vi "HFRR ADV v016 new software.vi"() -> ()   [LabVIEW 2025] (continued)
                n3061 = local write "Numeric 10"(w4047) -> ()
              }
              frame #1 {
                n3062 = local read "S.NO"() -> (→"s.NO":string)
                n3063 = local read "String 29"() -> (w4051:string)
                n3064 = String To Path(string=w4051) -> (path=w4050:path)
                n3065 = Open/Create/Replace File "Open File"(file path (use dialog)=w4050) -> (refnum out=w4052:refnum<file>)  [unwired: 5 in, 2 out]
                n3066 = for {
                  N: 16 -> [_]
                  tunnel: w4052 -> [w4059]
                  i -> [w4055]
                  (unwired) TRUE ("line mode (F)")
                  n3067 = Read from Text File "Read File"(file (use dialog)=w4059) -> (text=w4053:string)  [unwired: 3 in, 3 out]
                  n3068 = Match Pattern(string=w4053, regular expression="(") -> (after substring=w4058:string)  [unwired: 1 in, 3 out]
                  n3069 = Match Pattern(string=w4058, regular expression=")") -> (before substring=w4054:string)  [unwired: 1 in, 3 out]
                  n3070 = case shown="1" w4055 {
                    tunnel: w4054 -> [w4060 w4061 _ _ w4062 w4063 w4064 w4066 w4068 w4070 w4072 w4074 w4076 w4078 _]
                    tunnel: w4053 -> [_ _ _ _ _ _ _ _ _ _ _ _ _ _ _]
                    frame 0 {
                      "TITTLE" <- w4060
                    }
                    frame 1 {
                      "Sample ID" <- w4061
                    }
                    frame 2 {
                    }
                    frame 3 {
                    }
                    frame 4 {
                      "Test Date" <- w4062
                    }
                    frame 5 {
                      "Tested by" <- w4063
                    }
                    frame 6 {
                      n3071 = Fract/Exp String To Number(string=w4064) -> (number=→"Humidity before test 2":dbl)  [unwired: 3 in, 1 out]
                    }
                    frame 7 {
                      n3072 = Fract/Exp String To Number(string=w4066) -> (number=→"Temperature before test 2":dbl)  [unwired: 3 in, 1 out]
                    }
                    frame 8 {
                      n3073 = Fract/Exp String To Number(string=w4068) -> (number=→"Humidity after test 2":dbl)  [unwired: 3 in, 1 out]
                    }
                    frame 9 {
                      n3074 = Fract/Exp String To Number(string=w4070) -> (number=→"Temperature after test 2":dbl)  [unwired: 3 in, 1 out]
                    }
                    frame 10 {
                      n3075 = Fract/Exp String To Number(string=w4072) -> (number=→"MWSD 2":dbl)  [unwired: 3 in, 1 out]
                    }
                    frame 11 {
                      n3076 = Fract/Exp String To Number(string=w4074) -> (number=→"AVP 2":dbl)  [unwired: 3 in, 1 out]
                    }
                    frame 12 {
                      n3077 = Fract/Exp String To Number(string=w4076) -> (number=→"HCF 2":dbl)  [unwired: 3 in, 1 out]
                    }
                    frame 13 {
                      n3078 = Fract/Exp String To Number(string=w4078) -> (number=→"WS1.4 2":dbl)  [unwired: 3 in, 1 out]
                    }
                    frame 14, Default {
                    }
                  }
                }
              }
              frame #2 {
              }
            }
            n3079 = local write "OK Button 16"(FALSE ("OK Button 13")) -> ()
          }
        }
        n3080 = Index Array(array=w3722, index="Select Printer 3") -> (element=w3724:string)
        "Selected Printer" <- w3724
        n3081 = case shown="True" w3719 {
          frame False {
          }
          frame True {
            n3082 = flat-sequence {
              frame #0 {
              }
              frame #1 {
                n3083 = Wait (ms)(milliseconds to wait=u32 100) -> ()  [unwired: 1 out]
              }
              frame #2 {
                n3084 = local write "OK Button 16"(FALSE ("Print 3")) -> ()
              }
            }
          }
        }
        n3085 = case shown="True" "Print" {
          tunnel: w3724 -> [_ w4016]
          frame False {
          }
          frame True {
            (unwired) i16 6 ("width (-)")
            (unwired) "TESTED BY : "
            (unwired) "TESTED DATE :"
            (unwired) "SAMPLE ID : "
            (unwired) "SAMPLE DESIGN : "
            w3974 = "\r"
            w3991 = "\r"
            # "add image"
            n3086 = local read "Sample ID"() -> (w3964:string)
            n3087 = local read "Tested by"() -> (w3967:string)
            n3088 = local read "String 34"() -> (w3954:string)
            n3089 = local read "String 45"() -> (w3934:string)
            n3090 = local read "String 35"() -> (w3949:string)
            n3091 = local read "String 37"() -> (w3947:string)
            n3092 = local read "String 32"() -> (w3969:string)
            n3093 = local read "String 36"() -> (w3944:string)
            n3094 = local read "String 31"() -> (w3968:string)
            n3095 = local read "Test Date"() -> (w3965:string)
            n3096 = local read "String 33"() -> (w3970:string)
            n3097 = local read "String 38"() -> (w3940:string)
            n3098 = local read "String 39"() -> (w3937:string)
            n3099 = local write "Print"(FALSE ("Print FF")) -> ()
            n3100 = local read "S 39"() -> (w3952:string)
            n3101 = local read "S 38"() -> (w3959:string)
            n3102 = local read "Temperature before test 2"() -> (w3990:dbl)
            n3103 = local read "Temperature after test 2"() -> (w3980:dbl)
            n3104 = local read "Humidity before test 2"() -> (w4005:dbl)
            n3105 = local read "Humidity after test 2"() -> (w3989:dbl)
            n3106 = local read "MWSD 2"() -> (w3994:dbl)
            n3107 = local read "WS1.4 2"() -> (w3972:dbl)
            n3108 = Concatenate Strings("2)" ("string"), w3954) -> (w3955:string)
            n3109 = Concatenate Strings("3)" ("string"), w3952) -> (w3953:string)
            n3110 = Concatenate Strings("1)" ("string"), w3959) -> (w3958:string)
            n3111 = Concatenate Strings("4)" ("string"), w3949) -> (w3950:string)
            n3112 = Concatenate Strings("5)" ("string"), w3947) -> (w3946:string)
            n3113 = Concatenate Strings("6)" ("string"), w3944) -> (w3943:string)
            n3114 = Concatenate Strings("7)" ("string"), w3940) -> (w3941:string)
            n3115 = Concatenate Strings("8)" ("string"), w3937) -> (w3938:string)
            n3116 = local read "HCF 2"() -> (w3976:dbl)
            n3117 = local read "AVP 2"() -> (w3993:dbl)
            n3118 = local read "s.NO"() -> (w3935:string)
            n3119 = call <vilib>:"New Report.vi"("report type"=enum16{"Standard Report", "HTML"}."Standard Report") -> ("report out"=w4014:refnum<class "NI_report.lvclass">, "error out"=w4013:errorcluster)  [unwired: 13 in]
            n3120 = local read "TITTLE"() -> (w3966:string)
            n3121 = Concatenate Strings(w3991, w3934, w3935, w3991, w3969, w3964, w3991, w3968, w3965, w3991, w3970, w3967, w3991) -> (w3984:string)
            "test by" <- w3984
            n3122 = Number To Fractional String(number=w3990, width (-)=i16 6, precision (6)=i16 2) -> (F-format string=w3979:string)  [unwired: 1 in]
            n3123 = Number To Fractional String(number=w3989, width (-)=i16 6, precision (6)=i16 2) -> (F-format string=w3992:string)  [unwired: 1 in]
            n3124 = Number To Fractional String(number=w4005, width (-)=i16 6, precision (6)=i16 2) -> (F-format string=w4010:string)  [unwired: 1 in]
            n3125 = Number To Fractional String(number=w3994, width (-)=i16 6, precision (6)=i16 2) -> (F-format string=w3996:string)  [unwired: 1 in]
            n3126 = Number To Fractional String(number=w3980, width (-)=i16 6, precision (6)=i16 2) -> (F-format string=w3981:string)  [unwired: 1 in]
            n3127 = Number To Fractional String(number=w3993, width (-)=i16 6, precision (6)=i16 2) -> (F-format string=w3995:string)  [unwired: 1 in]
            n3128 = Number To Fractional String(number=w3976, width (-)=i16 6, precision (6)=i16 2) -> (F-format string=w3975:string)  [unwired: 1 in]
            n3129 = Number To Fractional String(number=w3972, precision (6)=i16 2) -> (F-format string=w3971:string)  [unwired: 2 in]
            n3130 = call-dynamic "Set Report Header Text.vi"("report in"=w4014, "center header text"=w3966, "error in (no error)"=w4013) -> ("report out"=w3985:refnum<class "NI_report.lvclass">, "error out"=w3986:errorcluster)  [unwired: 11 in]
            n3131 = Concatenate Strings(w3974, w3958, w4010, w3974, w3955, w3979, w3974, w3953, w3992, w3974, w3950, w3981, w3974, w3946, w3996, w3974, w3943, w3995, w3974, w3941, w3975, w3974, w3938, w3971) -> (w3962:string)
            "export 2" <- w3962
            n3132 = call-poly <vilib>:"Append Report Text.vi"("report in"=w3985, "text"=w3984, "error in (no error)"=w3986) -> ("report out"=w3988:refnum<class "NI_report.lvclass">, "error out"=w3987:errorcluster)  [unwired: 9 in, 2 out]
            n3133 = local read "test by"() -> (w3961:string)
            n3134 = local read "TITTLE"() -> (w3963:string)
            n3135 = call-poly <vilib>:"Append Report Text.vi"("report in"=w3988, "error in (no error)"=w3987) -> ("report out"=w4009:refnum<class "NI_report.lvclass">, "error out"=w4007:errorcluster)  [unwired: 10 in, 2 out]
            n3136 = Concatenate Strings(w3963, w3962, w3961) -> (→"output":string)
            n3137 = call-poly <vilib>:"Append Report Text.vi"("report in"=w4009, "text"=w3962, "error in (no error)"=w4007) -> ("report out"=w4008:refnum<class "NI_report.lvclass">, "error out"=w4006:errorcluster)  [unwired: 9 in, 2 out]
            n3138 = call-dynamic "Print Report.vi"("report in"=w4008, "printer name (default)"=w4016, "error in (no error)"=w4006) -> ("report out"=w4018:refnum<class "NI_report.lvclass">, "error out"=w4019:errorcluster)  [unwired: 11 in]
            n3139 = call-dynamic "Dispose Report.vi"("report in"=w4018, "error in (no error)"=w4019) -> ()  [unwired: 13 in, 1 out]
          }
        }
        n3140 = case shown="True" "Print 2" {
          frame False {
          }
          frame True {
            n3141 = flat-sequence {
              frame #0 {
                n3142 = local read "s.NO"() -> (→"s.NO 2":string)
                n3143 = Wait (ms)(milliseconds to wait=u32 20) -> ()  [unwired: 1 out]
                n3144 = local read "Sample ID  3"() -> (→"Sample ID  6":string)
                n3145 = local read "Sample ID  4"() -> (→"Sample ID  7":string)
                n3146 = local read "Sample ID"() -> (→"Sample ID  2":string)
                n3147 = local read "Tested by"() -> (→"Tested by 2":string)
                n3148 = local read "Test Date"() -> (→"Test Date 2":string)
                n3149 = local read "Humidity after test 3"() -> (→"Humidity after test 4":dbl)
                n3150 = local read "Ref A Test Date :"() -> (→"TITTLE 4":string)
                n3151 = local read "Temperature before test 3"() -> (w3841:dbl)
                n3152 = local read "Temperature before test 3"() -> (→"Temperature after test 5":dbl)
                n3153 = local read "Temperature after test 3"() -> (→"Temperature after test 4":dbl)
                n3154 = local read "Humidity before test 3"() -> (→"Humidity before test 4":dbl)
                n3155 = local write "Temperature before test 3"(w3841) -> ()
                n3156 = local read "image data"() -> (w3832:T16)
                n3157 = String To Path(string="C:\\LAB-IQ\\im\\Temp_resized.jpg") -> (path=w3833:path)
                "path 2" <- w3833
                n3158 = call <vilib>:"Write JPEG File.vi"("image data"=w3832, "path to JPEG file"=w3833) -> ()  [unwired: 8 in, 2 out]
                "Ref A Test Date :" <- "Ref A Test Date :"
                "Ref B Test Date :" <- "Ref B Test Date :"
                "Ref B Scar Value :" <- "Ref B Scar Value :"
                "Ref A Scar Value :" <- "Ref A Scar Value :"
              }
              frame #1 {
                (unwired) HTML_Report_Image_Alignment."MIDDLE" ("alignment (default)")
                w3869 = u16 0 items=["portrait", "landscape"] ("orientation (portrait)")
                (unwired) HTML_Report_Image_Alignment."ABSMIDDLE" ("alignment (default)")
                (unwired) "TESTED BY : "
                (unwired) "TESTED DATE :"
                (unwired) "SAMPLE ID : "
                (unwired) "SAMPLE DESIGN : "
                w3902 = "\r"
                # "add image"
                n3159 = Wait (ms)(milliseconds to wait=u32 20) -> ()  [unwired: 1 out]
                n3160 = local read "Sample ID  2"() -> (w3895:string)
                n3161 = local read "Wear Scar X"() -> (w3867:dbl)
                "Length ( microns ) 2" <- w3867
                n3162 = local read "Wear Scar Y"() -> (w3866:dbl)
                "Wear Scar Y ( microns ) :" <- w3866
                n3163 = local read "Test Date 2"() -> (w3896:string)
                n3164 = local read "Tested by 2"() -> (w3897:string)
                n3165 = local read "String 46"() -> (w3893:string)
                n3166 = local read "String 48"() -> (w3899:string)
                n3167 = local read "String 47"() -> (w3898:string)
                n3168 = local read "String 49"() -> (w3900:string)
                n3169 = local read "String 10"() -> (w3853:string)
                n3170 = local read "s.NO 2"() -> (w3894:string)
                n3171 = Add(x=w3867, y=w3866) -> (x+y=w3865:dbl)
                n3172 = call <vilib>:"New Report.vi"("report type"=enum16{"Standard Report", "HTML"}."HTML") -> ("report out"=w3873:refnum<class "NI_report.lvclass">, "error out"=w3871:errorcluster)  [unwired: 13 in]
                n3173 = Concatenate Strings(w3902, w3893, w3894, w3902, w3899, w3895, w3902, w3898, w3896, w3902, w3900, w3897, w3902) -> (→"test by 2":string)
                n3174 = Concatenate Strings("C:\\LAB-IQ\\Data\\" ("string"), w3853, ".jpg" ("string")) -> ()  [unwired: 1 out]
                n3175 = Divide(x=w3865, y=2.0) -> (x/y=→"Mean Wear ( microns) :":dbl)
                n3176 = call-dynamic "Set Report Orientation.vi"("report in"=w3873, "orientation (portrait)"=w3869, "error in (no error)"=w3871) -> ("report out"=w3872:refnum<class "NI_report.lvclass">, "error out"=w3870:errorcluster)  [unwired: 11 in]
                n3177 = for {
                  N: 5 -> [_]
                  tunnel: w3872 -> [w3923]
                  tunnel: [w3922] -> w3851
                  tunnel: w3870 -> [w3921]
                  tunnel: [w3920] -> w3850
                  n3178 = call-dynamic "Set Report Tab Width.vi"("report in"=w3923, "error in (no error)"=w3921) -> ("report out"=w3922:refnum<class "NI_report.lvclass">, "error out"=w3920:errorcluster)  [unwired: 12 in]
                }
                n3179 = local read "TITTLE"() -> (w3868:string)
                n3180 = call-dynamic "Set Report Header Text.vi"("report in"=w3851, "center header text"=w3868, "error in (no error)"=w3850) -> ("report out"=w3889:refnum<class "NI_report.lvclass">, "error out"=w3888:errorcluster)  [unwired: 11 in]
                n3181 = for {
                  N: 1 -> [_]
                  tunnel: [w3927] -> w3875
                  tunnel: [w3926] -> w3874
                  tunnel: w3889 -> [w3925]
                  tunnel: w3888 -> [w3924]
                  n3182 = call-dynamic "New Report Line.vi"("report in"=w3925, "error in (no error)"=w3924) -> ("report out"=w3927:refnum<class "NI_report.lvclass">, "error out"=w3926:errorcluster)  [unwired: 12 in]
                }
                n3183 = for {
                  N: 2 -> [_]
                  tunnel: [w3919] -> w3881
                  tunnel: [w3918] -> w3880
                  tunnel: w3875 -> [w3917]
                  tunnel: w3874 -> [w3916]
                  n3184 = call-dynamic "New Report Line.vi"("report in"=w3917, "error in (no error)"=w3916) -> ("report out"=w3919:refnum<class "NI_report.lvclass">, "error out"=w3918:errorcluster)  [unwired: 12 in]
                }
                n3185 = for {
                  N: 25 -> [_]
                  tunnel: w3881 -> [w3915]
                  tunnel: w3880 -> [w3913]
                  tunnel: [w3914] -> w3884
                  tunnel: [w3912] -> w3883
                  n3186 = call-dynamic "Set Report Tab Width.vi"("report in"=w3915, "error in (no error)"=w3913) -> ("report out"=w3914:refnum<class "NI_report.lvclass">, "error out"=w3912:errorcluster)  [unwired: 12 in]
                }
                n3187 = control-ref of="Tab Control 9"() -> (w3879:refnum<vi>)
                n3188 = call-dynamic "Append Control Image to Report.vi"("report in"=w3884, "alignment (default)"=HTML_Report_Image_Alignment."ABSMIDDLE", "ctrl reference"=w3879, "error in (no error)"=w3883) -> ("report out"=w3878:refnum<class "NI_report.lvclass">, "error out"=w3877:errorcluster)  [unwired: 8 in, 2 out]
                n3189 = for {
                  N: 3 -> [_]
                  tunnel: [w3911] -> w3862
                  tunnel: [w3910] -> w3861
                  tunnel: w3878 -> [w3909]
                  tunnel: w3877 -> [w3908]
                  n3190 = call-dynamic "New Report Line.vi"("report in"=w3909, "error in (no error)"=w3908) -> ("report out"=w3911:refnum<class "NI_report.lvclass">, "error out"=w3910:errorcluster)  [unwired: 12 in]
                }
                n3191 = for {
                  N: 100 -> [_]
                  tunnel: w3862 -> [w3907]
                  tunnel: w3861 -> [w3905]
                  tunnel: [w3906] -> w3858
                  tunnel: [w3904] -> w3856
                  n3192 = call-dynamic "Set Report Tab Width.vi"("report in"=w3907, "error in (no error)"=w3905) -> ("report out"=w3906:refnum<class "NI_report.lvclass">, "error out"=w3904:errorcluster)  [unwired: 12 in]
                }
                n3193 = String To Path(string="C:\\LAB-IQ\\im\\Temp_resized.jpg") -> (path=w3848:path)
                n3194 = call-poly <vilib>:"Append Image to Report.vi"("report in"=w3858, "path or URL of image"=w3848, "error in (no error)"=w3856) -> ("report out"=w3857:refnum<class "NI_report.lvclass">, "error out"=w3855:errorcluster)  [unwired: 9 in, 2 out]
                n3195 = call-poly <vilib>:"Open HTML Report in Browser.vi"("report in"=w3857, "error in (no error)"=w3855) -> ("report out"=w3892:refnum<class "NI_report.lvclass">, "error out"=w3891:errorcluster)  [unwired: 11 in, 1 out]
                n3196 = call-dynamic "Dispose Report.vi"("report in"=w3892, "error in (no error)"=w3891) -> ()  [unwired: 13 in, 1 out]
              }
              frame #2 {
              }
              frame #3 {
                n3197 = disable-structure shown="Disabled" {
                  frame Disabled {
                    n3198 = local read "String 10"() -> (w3932:string)
                    n3199 = Concatenate Strings("C:\\LAB-IQ-NXT\\Data\\" ("string"), w3932, ".jpg" ("string")) -> (w3930:string)
                    n3200 = String To Path(string=w3930) -> (path=w3929:path)
                    n3201 = Delete(path (use dialog)=w3929) -> ()  [unwired: 4 in, 3 out]
                  }
                  frame Enabled {
                  }
                }
                n3202 = local write "Print 2"(FALSE ("Print")) -> ()
              }
            }
          }
        }
      }
    }
    n3203 = property on="SetTemp" class="DigNum (strict)"("Disabled"=w1868) -> ()  [unwired: 2 in, 2 out]
    n3204 = Multiply(x=w1858, y=w1860) -> (x*y=w1859:dbl)
    n3205 = local read "MWSD"() -> (w1857:dbl)
    n3206 = Add(x=w1859, y=w1857) -> (x+y=→"WS1.4":dbl)
    n3207 = Wait (ms)(milliseconds to wait=u32 50) -> ()  [unwired: 1 out]
    n3208 = Wait (ms)(milliseconds to wait=u32 50) -> ()  [unwired: 1 out]
    n3209 = local read "Quit"() -> (w1856:bool)
  }
  n3210 = VISA Close(VISA resource name=w52, error in (no error)=w51) -> (error out=w49:errorcluster)
  n3211 = call <vilib>:"Clear Errors.vi"("error in (no error)"=w49) -> ()  [unwired: 5 in, 2 out]
  n3212 = VISA Close(VISA resource name=w37, error in (no error)=w36) -> ()  [unwired: 1 out]
  n3213 = while {
    tunnel: [w4093] -> w46
    shift-right: [w4086] -> _
    shift-left: 0.0 -> [w4089]
    shift-right: [w4085] -> _
    shift-left: 0.0 -> [w4088]
    shift-right: [w4084] -> _
    shift-left: 400.0 ("vc_cmd") -> [w4087]
    stop <- w4093 stop-if-true
    # "PID LOGIC"
    n3214 = local read "RUN"() -> (w4091:bool)
    n3215 = local read "Auto Start Temp"() -> (w4080:bool)
    n3216 = local read "Auto Start Test"() -> (w4090:bool)
    n3217 = local read "START TEMP"() -> (w4082:bool)
    n3218 = And(x=w4080, y=w4090) -> (x .and. y?=w4081:bool)
    n3219 = Or(x=w4091, y=w4081) -> (x .or. y?=w4092:bool)
    n3220 = And(x=w4092, y=w4082) -> (x .and. y?=w4083:bool)
    n3221 = Wait (ms)(milliseconds to wait=u32 20) -> ()  [unwired: 1 out]
    n3222 = case shown="True" w4083 {
      tunnel: [400.0 ("out_vc_cmd") w4113] -> w4084
      tunnel: [w4096 w4115] -> w4085
      tunnel: [w4096 w4114] -> w4086
      tunnel: w4089 -> [_ w4104]
      tunnel: w4088 -> [_ w4103]
      tunnel: w4087 -> [_ w4102]
      frame False {
        w4096 = 0.0 ("error_out")
      }
      frame True {
        n3223 = local read "Set Strk"() -> (w4099:dbl)
        n3224 = local read "LVDT STROKE"() -> (w4097:dbl)
        n3225 = Add(x=w4099, y="Add up Stroke") -> (x+y=w4100:dbl)
        n3226 = formula code="// Zero-Hardcode Explicit Positional-Form PID Engine\n// Inputs: target_stroke, measured_stroke, dt, prev_error, integral_accumulator_in, prev_vc_cmd\n//         kp, ki, kd, max_step_change, max_amplitude, min_amplitude, startup_cmd\n// Outputs: vc_cmd, error_out, out_error, integral_accumulator_out, out_vc_cmd\n\n// 1. Calculate Tracking Error\nfloat current_error = target_stroke - measured_stroke;\nerror_out = current_error;\n\n// 2. Compute Proportional Term\nfloat p_term = kp * current_error;\n\n// 3. Compute Derivative Term\nfloat d_term = 0.0;\nif (dt > 0.0) {\n    d_term = kd * ((current_error - prev_error) / dt);\n}\n\n// 4. Update and Accumulate Integral Term\nfloat current_integral = integral_accumulator_in + (current_error * dt);\nfloat i_term = ki * current_integral;\n\n// 5. Calculate Ideal Target Command\nfloat ideal_command = startup_cmd + p_term + i_term + d_term;\n\n// 6. Anti-Windup Protection (Back-calculation method)\nif (ideal_command > max_amplitude) {\n    float excess = ideal_command - max_amplitude;\n    if (ki > 0.0) {\n        current_integral -= excess / ki;\n    }\n    ideal_command = max_amplitude;\n} else if (ideal_command < min_amplitude) {\n    float excess = ideal_command - min_amplitude;\n    if (ki > 0.0) {\n        current_integral -= excess / ki;\n    }\n    ideal_command = min_amplitude;\n}\n\n// 7. Apply Loop Rate Limiting (Protects voice coil from large voltage steps)\nfloat raw_adjustment = ideal_command - prev_vc_cmd;\n\nif (raw_adjustment > max_step_change) {\n    raw_adjustment = max_step_change;\n} else if (raw_adjustment < -max_step_change) {\n    raw_adjustment = -max_step_change;\n}\n\nfloat next_vc_cmd = prev_vc_cmd + raw_adjustment;\n\n// Final Output Safety Safeguard Clamping\nif (next_vc_cmd > max_amplitude) {\n    next_vc_cmd = max_amplitude;\n} else if (next_vc_cmd < min_amplitude) {\n    next_vc_cmd = min_amplitude;\n}\n\n// 8. Map to Shift Registers for memory persistence\nvc_cmd = next_vc_cmd;\nout_error = current_error;                     \nintegral_accumulator_out = current_integral;  \nout_vc_cmd = next_vc_cmd;"("target_stroke"=w4100, "measured_stroke"=w4097, "dt"="dt", "integral_accumulator_in"=w4103, "prev_error"=w4104, "prev_vc_cmd"=w4102, "kp"="kp", "ki"="ki", "kd"="kd", "max_step_change"="max_step_change", "max_amplitude"="max_amplitude", "min_amplitude"="min_amplitude", "startup_cmd"="startup_cmd") -> ("vc_cmd"=w4119:dbl, "out_error"=w4114:dbl, "integral_accumulator_out"=w4115:dbl, "out_vc_cmd"=w4113:dbl)  [unwired: 1 out]
        "output Vpp" <- w4119
        n3227 = Number To Fractional String(number=w4119, precision (6)=i16 1) -> (F-format string=w4117:string)  [unwired: 2 in]
        n3228 = Concatenate Strings("DAC;" ("string"), w4117) -> (w4101:string)
        n3229 = local write "Command"(w4101) -> ()
        "prev_error" <- w4104
        "integral_accumulator_in" <- w4103
        "prev_vc_cmd" <- w4102
      }
    }
    n3230 = local read "Quit"() -> (w4093:bool)
  }
  n3231 = Or(x=w42, y=w41) -> (x .or. y?=w43:bool)
  n3232 = Or(x=w39, y=w43) -> (x .or. y?=w48:bool)
  n3233 = control-ref of="new picture"() -> ()  [unwired: 1 out]
  n3234 = Or(x=w54, y=w48) -> (x .or. y?=w45:bool)
  n3235 = Or(x=w45, y=w46) -> (x .or. y?=w40:bool)
  n3236 = while {
    tunnel: [w4120] -> w53
    i -> [w4127]
    stop <- w4120 stop-if-true
    n3237 = local read "Quit"() -> (w4120:bool)
    n3238 = Equal To 0?(x=w4127) -> (x = 0?=w4125:bool)
    n3239 = call "Elapsed Time3"("Time Target (s)"=45.0, "Auto Reset"=TRUE) -> ("Time has Elapsed"=w4124:bool)  [unwired: 10 in, 7 out]
    n3240 = Wait (ms)(milliseconds to wait=u32 50) -> ()  [unwired: 1 out]
    n3241 = Or(x=w4124, y=w4125) -> (x .or. y?=w4126:bool)
    n3242 = case shown="True" w4126 {
      frame False {
      }
      frame True {
        n3243 = call <vilib>:"System Exec.vi"("run minimized? (F)"=TRUE, "error in (no error)"="error in (no error)", "command line"="powercfg.exe -change -monitor-timeout-ac 0") -> ("error out"=w4138:errorcluster)  [unwired: 5 in, 3 out]
        n3244 = call <vilib>:"System Exec.vi"("run minimized? (F)"=TRUE, "error in (no error)"=w4138, "command line"="powercfg.exe -change -disk-timeout-ac 0") -> ("error out"=w4137:errorcluster)  [unwired: 5 in, 3 out]
        n3245 = call <vilib>:"System Exec.vi"("run minimized? (F)"=TRUE, "error in (no error)"=w4137, "command line"="powercfg.exe -change -standby-timeout-ac 0") -> ("error out"=w4136:errorcluster)  [unwired: 5 in, 3 out]
        n3246 = call <vilib>:"System Exec.vi"("run minimized? (F)"=TRUE, "error in (no error)"=w4136, "command line"="powercfg.exe -change -hibernate-timeout-ac 0") -> ("error out"=w4135:errorcluster)  [unwired: 5 in, 3 out]
        n3247 = call <vilib>:"Simple Error Handler.vi"("error in (no error)"=w4135) -> ("error out"=w4141:errorcluster)  [unwired: 4 in, 4 out]
        n3248 = call <vilib>:"Clear Errors.vi"("error in (no error)"=w4141) -> ("error out"=→"error out":errorcluster)  [unwired: 5 in, 1 out]
      }
    }
  }
  n3249 = Compound Arithmetic op=OR(w56, w40, w53) -> (w55:bool)
  n3250 = flat-sequence {
    tunnel: w55 -> [_]
    tunnel: [w4143] -> w18
    tunnel: w18 -> [_]
    frame #0 {
      n3251 = call "CLOSE CONNECTION.vi"() -> ("error out"=w4143:errorcluster)  [unwired: 11 in]
    }
    frame #1 {
      n3252 = Quit LabVIEW(quit? (T)=TRUE) -> ()
      n3253 = local write "Quit"(FALSE ("EXIT")) -> ()
    }
  }
  n3254 = property on="Heater Button" class="Bool (strict)"("Visible"=TRUE) -> ()  [unwired: 2 in, 2 out]
  n3255 = disable-structure shown="Disabled" {
    disable-tunnel: _ -> [w4149 _]
    disable-tunnel: _ -> [w4146 _]
    disable-tunnel: _ -> [w4147 _]
    frame Disabled {
      n3256 = disable-structure shown="Disabled" {
        disable-tunnel: [w4156 _] -> w4148
        frame Disabled {
          n3257 = while {
            shift-right: [w4198] -> w4154
            shift-left: errorcluster {"status"=TRUE, "code"=0, "source"="Init"} ("error out") -> [w4163]
            shift-right: [w4197] -> w4153
            shift-left: _ -> [w4164]
            shift-right: [w4196] -> _
            shift-left: "" -> [w4195]
            tunnel: [w4157] -> w4156
            shift-right: ["Set Rh"] -> _
            shift-left: 0.0 ("Set Rh") -> [w4189]
            tunnel: [w4166] -> _
            i -> [w4166]
            stop <- w4157 stop-if-true
            n3258 = flat-sequence {
              tunnel: w4163 -> [w4201]
              tunnel: [w4201] -> w4162
              frame #0 {
                n3259 = Wait (ms)(milliseconds to wait=u32 200) -> ()  [unwired: 1 out]
              }
            }
            n3260 = local read "Com Port 3"() -> (w4165:refnum<visa-resource-name>)
            n3261 = local read "Humidity Str Rec"() -> (w4167:string)
            n3262 = Not Equal?(x="Set Rh", y=w4189) -> (x != y?=w4194:bool)
            n3263 = Number To Decimal String(number="Set Rh") -> (decimal integer string=w4192:string)  [unwired: 1 in]
            n3264 = Not Equal?(x=w4165, y=w4164) -> (x != y?=w4160:bool)
            n3265 = Concatenate Strings("#setPoint00" ("string"), w4192) -> (w4193:string)
            n3266 = case shown="False" w4194 {
              tunnel: w4193 -> [_ w4213]
              frame False {
                n3267 = local read "Humidity"() -> (w4210:bool)
                n3268 = case shown="True" w4210 {
                  frame False {
                    n3269 = local write "Humidity Str Send"("stop" ("Humidity Str Send")) -> ()
                  }
                  frame True {
                    n3270 = local write "Humidity Str Send"("start" ("Humidity Str Send")) -> ()
                  }
                }
              }
              frame True {
                n3271 = local write "Humidity Str Send"(w4213) -> ()
              }
            }
            n3272 = Or(x=w4160) -> (y=w4158:bool, x .or. y?=w4159:bool)
            n3273 = String Subset(string=w4167, offset (0)=7) -> (substring=w4182:string)  [unwired: 1 in]
            n3274 = Match Pattern(string=w4167, regular expression="?") -> (offset past match=w4185:i32)  [unwired: 1 in, 3 out]
            n3275 = Match Pattern(string=w4167, regular expression="v") -> (offset past match=w4188:i32)  [unwired: 1 in, 3 out]
            n3276 = case shown="True" w4159 {
              tunnel: w4162 -> [w4199 _]
              tunnel: [w4199 errorcluster {"status"=TRUE, "code"=0, "source"="Init"} ("error out")] -> w4161
              frame False {
              }
              frame True {
              }
            }
            n3277 = Equal?(x=w4185, y=-1) -> (x = y?=w4169:bool)
            n3278 = Match Pattern(string=w4182, regular expression="g") -> (after substring=w4183:string, offset past match=w4174:i32)  [unwired: 1 in, 2 out]
            n3279 = Match Pattern(string=w4182, regular expression="y") -> (after substring=w4181:string, offset past match=w4175:i32)  [unwired: 1 in, 2 out]
            n3280 = Greater?(x=w4175, y=w4174) -> (0:w4180:bool)
            n3281 = Greater Or Equal To 0?(x=w4175) -> (x >= 0?=w4172:bool)
            n3282 = Greater Or Equal To 0?(x=w4174) -> (x >= 0?=w4173:bool)
            n3283 = Or(x=w4172, y=w4173) -> (x .or. y?=w4171:bool)
            n3284 = Greater Or Equal To 0?(x=w4188) -> (x >= 0?=w4170:bool)
            n3285 = Select(t=w4181, s=w4180, f=w4183) -> (s? t:f=w4176:string)
            n3286 = case shown="Error" w4161 {
              selector: w4161 -> [w4226 w4272]
              tunnel: [w4224 w4265] -> w4198
              tunnel: w4164 -> [w4227 w4271]
              tunnel: [w4225 w4274] -> w4197
              tunnel: w4195 -> [w4214 w4273]
              tunnel: [w4221 w4273] -> w4196
              frame No Error {
                n3287 = call "Elapsed Time7"() -> ("Time has Elapsed"=w4220:bool)  [unwired: 12 in, 7 out]
                n3288 = Not Equal?(x="Humidity Str Send", y=w4214) -> (x != y?=w4216:bool)
                n3289 = Or(x=w4216, y=w4220) -> (x .or. y?=w4219:bool)
                n3290 = Select(t="Humidity Str Send", s=w4216, f="vals" ("regular expression")) -> (s? t:f=w4215:string)
                n3291 = Or(x=w4219, y="Send") -> (x .or. y?=w4223:bool)
                n3292 = case shown="True" w4223 {
                  tunnel: [w4230 w4235] -> w4224
                  tunnel: w4227 -> [w4229 w4243]
                  tunnel: w4226 -> [w4230 w4242]
                  tunnel: [w4229 w4236] -> w4225
                  tunnel: w4215 -> [_ w4241]
                  tunnel: [w4228 w4232] -> w4221
                  tunnel: "Humidity Str Send" -> [_ w4233]
                  tunnel: w4216 -> [_ w4234]
                  tunnel: w4214 -> [w4228 w4231]
                  frame False {
                  }
                  frame True {
                    n3293 = flat-sequence {
                      tunnel: w4243 -> [w4251]
                      tunnel: w4242 -> [w4250]
                      tunnel: w4241 -> [w4247]
                      tunnel: [w4249] -> w4240
                      tunnel: [w4248] -> w4239
                      tunnel: w4240 -> [w4254]
                      tunnel: w4239 -> [w4253]
                      tunnel: [w4254] -> w4238
                      tunnel: [w4253] -> w4237
                      tunnel: w4238 -> [w4261]
                      tunnel: w4237 -> [w4260]
                      tunnel: [w4259] -> w4236
                      tunnel: [w4258] -> w4235
                      frame #0 {
                        n3294 = local write "Ser Led"(TRUE ("Boolean 4")) -> ()
                        n3295 = Concatenate Strings(w4247, "\r") -> (w4246:string)
                        n3296 = VISA Write(VISA resource name=w4251, write buffer=w4246, error in (no error)=w4250) -> (VISA resource name out=w4249:refnum<visa-resource-name>, error out=w4248:errorcluster)  [unwired: 1 out]
                      }
                      frame #1 {
                        n3297 = Wait (ms)(milliseconds to wait="wait") -> ()  [unwired: 1 out]
                      }
                      frame #2 {
                        w4256 = FALSE ("Send")
                        n3298 = property class="Instr"(reference=w4261, error in=w4260) -> (reference out=w4262:refnum<visa-resource-name>, error out=w4263:errorcluster, "Serial Settings:Number of Bytes at Serial Port"=w4255:u32)
                        n3299 = local write "Send"(w4256) -> ()
                        n3300 = local write "Ser Led"(w4256) -> ()
                        n3301 = VISA Read(VISA resource name=w4262, byte count=w4255, error in (no error)=w4263) -> (VISA resource name out=w4259:refnum<visa-resource-name>, read buffer=→"Humidity Str Rec":string, error out=w4258:errorcluster)  [unwired: 1 out]
                      }
                    }
                    n3302 = Select(t=w4233, s=w4234, f=w4231) -> (s? t:f=w4232:string)
                  }
                }
              }
              frame Error {
                w4279 = u16 0 items=["None"=0, "XON/XOFF"=1, "RTS/CTS"=2, "DTR/DSR"=4] ("flow control")
                w4275 = u16 0 items=["None", "Odd", "Even", "Mark", "Space"] ("parity")
                w4278 = u16 10 items=["1.0"=10, "1.5"=15, "2.0"=20] ("stop bits")
                n3303 = VISA Close(VISA resource name=w4271, error in (no error)=w4272) -> (error out=w4270:errorcluster)
                n3304 = local write "humid"("" ("humid")) -> ()
                n3305 = local write "Humidity Str Rec"("" ("Humidity Str Rec")) -> ()
                n3306 = call <vilib>:"Clear Errors.vi"("error in (no error)"=w4270) -> ("error out"=w4269:errorcluster)  [unwired: 5 in, 1 out]
                n3307 = local read "Com Port 3"() -> (w4268:refnum<visa-resource-name>)
                n3308 = call-poly "VISA Configure Serial Port"("VISA resource name"=w4268, "timeout (10sec)"=u32 1000, "termination char\n(0xA = '\\n' = LF)"=u8 10 ("termination char\n(0xA = '\\n' = LF)"), "Enable Termination\nChar (T)"=FALSE ("Enable Termination Char (T)"), "data bits (8)"=u16 8 ("data bits"), "parity (0:none)"=w4275, "error in (no error)"=w4269, "stop bits (10: 1 bit)"=w4278, "flow control (0:none)"=w4279) -> ("VISA resource name out"=w4274:refnum<visa-resource-name>, "baud rate (9600)"=w4266:u32, "error out"=w4265:errorcluster)  [unwired: 4 in]
              }
            }
            n3309 = Compound Arithmetic op=AND(w4170, w4169, w4171) -> (w4168:bool)
            n3310 = case shown="True" w4168 {
              tunnel: w4167 -> [_ _]
              tunnel: w4176 -> [_ w4206]
              frame False {
              }
              frame True {
                w4204 = " " ("regular expression")
                n3311 = Match Pattern(string=w4206, regular expression=" ") -> (after substring=w4208:string)  [unwired: 1 in, 3 out]
                n3312 = Match Pattern(string=w4208, regular expression=w4204) -> (before substring=→"humid":string, after substring=w4205:string)  [unwired: 1 in, 2 out]
                n3313 = Match Pattern(string=w4205, regular expression=w4204) -> (before substring=→"temp_@Rh sensor":string)  [unwired: 1 in, 3 out]
              }
            }
            n3314 = local read "Quit"() -> (w4157:bool)
          }
          n3315 = VISA Close(VISA resource name=w4153, error in (no error)=w4154) -> (error out=w4150:errorcluster)
          n3316 = call <vilib>:"Clear Errors.vi"("error in (no error)"=w4150) -> ()  [unwired: 5 in, 2 out]
        }
        frame Enabled {
        }
      }
    }
    frame Enabled {
    }
  }
  n3317 = while {
    tunnel: [w4286] -> _
    i -> [w4286]
    stop <- w4282 stop-if-true
    # "Langauage selection"
    n3318 = Equal?(x="Lan flag", y=22.0) -> ()  [unwired: 1 out]
    n3319 = disable-structure shown="Disabled" {
      frame Disabled {
        n3320 = stacked-sequence {
          frame #0 {
            n3321 = case shown="\"Russian\"" "Language Selection" {
              tunnel: [0 1] -> w4288
              frame "English", Default {
              }
              frame "Russian" {
              }
            }
            n3322 = for {
              N: 130 -> [_]
              tunnel: "Table" -> [w4297]
              tunnel: w4288 -> [w4296]
              i -> [w4295]
              n3323 = Index Array(array=w4297, index (row)=w4295, index (col)=w4296) -> (element=w4294:string)
              n3324 = case shown="123" w4295 {
                tunnel: w4294 -> [w4298 w4299 _ w4300 w4301 w4302 w4303 w4304 w4305 w4306 w4307 w4308 w4309 w4310 w4311 w4312 w4313 w4314 w4315 w4316 w4317 w4318 w4319 w4320 w4321 w4322 w4323 w4324 w4325 _ _ w4326 w4327 w4328 w4329 w4330 w4331 w4340 w4347 w4354 w4361 w4365 w4368 w4371 w4373 w4375 w4376 w4377 w4378 w4379 w4380 w4381 w4382 w4383 w4384 w4385 w4386 w4387 w4388 w4389 w4390 w4391 w4392 w4393 w4394 w4395 w4396 w4397 w4398 w4399 w4400 w4401 w4402 w4403 w4404 w4405 w4406 w4407 w4408 w4409 w4410 w4411 w4412 w4413 w4414 w4415 w4416 w4417 w4418 w4419 w4420 w4421 w4422 w4423 w4424 w4425 w4426 w4427 w4428 w4429 w4430 w4431 w4432 w4433 w4434 _ w4435 w4436 w4437 w4438 w4439 w4440 w4441 w4442 w4443 w4444 w4445 w4446 w4447 _ w4448 w4449 w4450 w4451 w4452 w4453 _]
                frame 0 {
                  n3325 = local write "S"(w4298) -> ()
                }
                frame 1 {
                  n3326 = local write "S 2"(w4299) -> ()
                }
                frame 2 {
                }
                frame 3 {
                  n3327 = local write "S 4"(w4300) -> ()
                }
                frame 4 {
                  n3328 = property on="FILE" class="Str"("Caption.Text"=w4301) -> ()  [unwired: 2 in, 2 out]
                }
                frame 5 {
                  n3329 = property on="Fuel Discription :" class="Str"("Caption.Text"=w4302) -> ()  [unwired: 2 in, 2 out]
                }
                frame 6 {
                  n3330 = property on="Remarks :" class="Str"("Caption.Text"=w4303) -> ()  [unwired: 2 in, 2 out]
                }
                frame 7 {
                  n3331 = property on="Save & Continue" class="Bool (strict)"("Boolean Text.Text"=w4304) -> ()  [unwired: 2 in, 2 out]
                }
                frame 8 {
                }
                frame 9 {
                  n3332 = property on="Set Hz" class="DigNum (strict)"("Caption.Text"=w4306) -> ()  [unwired: 2 in, 2 out]
                }
                frame 10 {
                  "String 3" <- w4307
                }
                frame 11 {
                  n3333 = property on="NORMAL LOAD" class="DigNum (strict)"("Caption.Text"=w4308) -> ()  [unwired: 2 in, 2 out]
                }
                frame 12 {
                  "String 5" <- w4309
                }
                frame 13 {
                  n3334 = property on="Set Temp" class="DigNum (strict)"("Caption.Text"=w4310) -> ()  [unwired: 2 in, 2 out]
                }
                frame 14 {
                  n3335 = local write "S 15"(w4311) -> ()
                }
                frame 15 {
                  n3336 = property on="Set Rh" class="DigNum (strict)"("Caption.Text"=w4312) -> ()  [unwired: 2 in, 2 out]
                }
                frame 16 {
                  "String 13" <- w4313
                  "String 26" <- w4313
                }
                frame 17 {
                  n3337 = local write "S 18"(w4314) -> ()
                }
                frame 18 {
                  "String 17" <- w4315
                }
                frame 19 {
                  n3338 = property on="test time" class="DigNum (strict)"("Caption.Text"=w4316) -> ()  [unwired: 2 in, 2 out]
                }
                frame 20 {
                  "String 18" <- w4317
                  "String 22" <- w4317
                }
                frame 21 {
                  n3339 = property on="Elapsed time" class="DigNum (strict)"("Caption.Text"=w4318) -> ()  [unwired: 2 in, 2 out]
                }
                frame 22 {
                  n3340 = property on="Samplingtime 2" class="DigNum (strict)"("Caption.Text"=w4319) -> ()  [unwired: 2 in, 2 out]
                }
                frame 23 {
                  "String 21" <- w4320
                }
                frame 24 {
                  n3341 = property on="Countdown" class="DigNum (strict)"("Caption.Text"=w4321) -> ()  [unwired: 2 in, 2 out]
                }
                frame 25 {
                  n3342 = property on="Countdown 2" class="DigNum (strict)"("Caption.Text"=w4322) -> ()  [unwired: 2 in, 2 out]
                }
                frame 26 {
                  n3343 = property on="Engage" class="Bool (strict)"("Boolean Text.Text"=w4323) -> ()  [unwired: 2 in, 2 out]
                }
                frame 27 {
                  n3344 = property on="Boolean  4" class="Bool (strict)"("Boolean Text.Text"=w4324) -> ()  [unwired: 2 in, 2 out]
                }
                frame 28 {
                  n3345 = property on="Test \nStatus" class="Bool (strict)"("Boolean Text.Text"=w4325) -> ()  [unwired: 2 in, 2 out]
                }
                frame 29 {
                }
                frame 30 {
                }
                frame 31 {
                }
                frame 32 {
                  n3346 = property on="RSTCOF" class="Bool"("Boolean Text.Text"=w4327) -> ()  [unwired: 2 in, 2 out]
                  n3347 = property on="RST FF" class="Bool"("Boolean Text.Text"=w4327) -> ()  [unwired: 2 in, 2 out]
                  n3348 = property on="RST TEMP" class="Bool"("Boolean Text.Text"=w4327) -> ()  [unwired: 2 in, 2 out]
                  n3349 = property on="RSTV1 3" class="Bool"("Boolean Text.Text"=w4327) -> ()  [unwired: 2 in, 2 out]
                  n3350 = property on="rstv2" class="Bool"("Boolean Text.Text"=w4327) -> ()  [unwired: 2 in, 2 out]
                  n3351 = property on="RSTV1 2" class="Bool"("Boolean Text.Text"=w4327) -> ()  [unwired: 2 in, 2 out]
                  n3352 = property on="RST CP" class="Bool"("Boolean Text.Text"=w4327) -> ()  [unwired: 2 in, 2 out]
                }
                frame 33 {
                  "S 61" <- w4328
                }
                frame 34 {
                  "String 23" <- w4329
                }
                frame 35 {
                  n3353 = property on="Rh Before" class="DigNum (strict)"("Caption.Text"=w4330) -> ()  [unwired: 2 in, 2 out]
                }
                frame 36 {
                  n3354 = Match Pattern(string=w4331, regular expression=",") -> (before substring=→"bs":string, after substring=→"as":string)  [unwired: 1 in, 2 out]
                  n3355 = property on="Rh After" class="DigNum (strict)"("Caption.Text"=w4331) -> ()  [unwired: 2 in, 2 out]
                }
                frame 37 {
                  n3356 = Match Pattern(string=w4340, regular expression=",") -> (before substring=w4339:string, after substring=w4338:string)  [unwired: 1 in, 2 out]
                  "bs" <- w4339
                  "as" <- w4338
                  n3357 = Concatenate Strings(w4339, w4338) -> (w4335:string)
                  n3358 = property on="Humidity before test 2" class="DigNum (strict)"("Caption.Text"=w4335) -> ()  [unwired: 2 in, 2 out]
                  n3359 = property on="Humidity before test" class="DigNum (strict)"("Caption.Text"=w4335) -> ()  [unwired: 2 in, 2 out]
                  n3360 = Concatenate Strings(w4335, "=" ("string")) -> (w4336:string)
                  n3361 = local write "S 38"(w4336) -> ()
                }
                frame 38 {
                  n3362 = Match Pattern(string=w4347, regular expression=",") -> (before substring=w4346:string, after substring=w4345:string)  [unwired: 1 in, 2 out]
                  "bs" <- w4346
                  "as" <- w4345
                  n3363 = Concatenate Strings(w4346, w4345) -> (w4342:string)
                  n3364 = property on="Humidity after test 2" class="DigNum (strict)"("Caption.Text"=w4342) -> ()  [unwired: 2 in, 2 out]
                  n3365 = Concatenate Strings(w4342, "=" ("string")) -> (w4344:string)
                  n3366 = property on="Humidity after test" class="DigNum (strict)"("Caption.Text"=w4342) -> ()  [unwired: 2 in, 2 out]
                  n3367 = local write "S 39"(w4344) -> ()
                }
                frame 39 {
                  n3368 = Match Pattern(string=w4354, regular expression=",") -> (before substring=w4353:string, after substring=w4352:string)  [unwired: 1 in, 2 out]
                  "bs" <- w4353
                  "as" <- w4352
                  n3369 = Concatenate Strings(w4353, w4352) -> (w4349:string)
                  n3370 = property on="Temperature before test 2" class="DigNum (strict)"("Caption.Text"=w4349) -> ()  [unwired: 2 in, 2 out]
                  n3371 = property on="Temperature before test" class="DigNum (strict)"("Caption.Text"=w4349) -> ()  [unwired: 2 in, 2 out]
                  n3372 = Concatenate Strings(w4349, "=" ("string")) -> (→"String 34":string)
                }
                frame 40 {
                  n3373 = Match Pattern(string=w4361, regular expression=",") -> (before substring=w4360:string, after substring=w4359:string)  [unwired: 1 in, 2 out]
                  "bs" <- w4360
                  "as" <- w4359
                  n3374 = Concatenate Strings(w4360, w4359) -> (w4356:string)
                  n3375 = property on="Temperature after test 2" class="DigNum (strict)"("Caption.Text"=w4356) -> ()  [unwired: 2 in, 2 out]
                  n3376 = Concatenate Strings(w4356, "=" ("string")) -> (→"String 35":string)
                  n3377 = property on="Temperature after test" class="DigNum (strict)"("Caption.Text"=w4356) -> ()  [unwired: 2 in, 2 out]
                }
                frame 41 {
                  n3378 = property on="AVP" class="DigNum (strict)"("Caption.Text"=w4365) -> ()  [unwired: 2 in, 2 out]
                  n3379 = property on="AVP 2" class="DigNum (strict)"("Caption.Text"=w4365) -> ()  [unwired: 2 in, 2 out]
                  n3380 = Concatenate Strings(w4365, "=" ("string")) -> (→"String 36":string)
                }
                frame 42 {
                  n3381 = property on="MWSD" class="DigNum (strict)"("Caption.Text"=w4368) -> ()  [unwired: 2 in, 2 out]
                  n3382 = property on="MWSD 2" class="DigNum (strict)"("Caption.Text"=w4368) -> ()  [unwired: 2 in, 2 out]
                  n3383 = Concatenate Strings(w4368, "=" ("string")) -> (→"String 37":string)
                }
                frame 43 {
                  n3384 = property on="HCF 2" class="DigNum (strict)"("Caption.Text"=w4371) -> ()  [unwired: 2 in, 2 out]
                  n3385 = property on="HCF" class="DigNum (strict)"("Caption.Text"=w4371) -> ()  [unwired: 2 in, 2 out]
                  n3386 = Concatenate Strings(w4371, "=" ("string")) -> (→"String 38":string)
                }
                frame 44 {
                  n3387 = Concatenate Strings(w4373, "=" ("string")) -> (→"String 39":string)
                  n3388 = property on="WS1.4 2" class="DigNum (strict)"("Caption.Text"=w4373) -> ()  [unwired: 2 in, 2 out]
                  n3389 = property on="WS1.4" class="DigNum (strict)"("Caption.Text"=w4373) -> ()  [unwired: 2 in, 2 out]
                }
                frame 45 {
                  n3390 = property on="Save Results" class="Bool (strict)"("Boolean Text.Text"=w4375) -> ()  [unwired: 2 in, 2 out]
                }
                frame 46 {
                  n3391 = local write "S 47"(w4376) -> ()
                }
                frame 47 {
                  n3392 = local write "S 48"(w4377) -> ()
                }
                frame 48 {
                  n3393 = local write "S 49"(w4378) -> ()
                }
                frame 49 {
                  n3394 = local write "S 50"(w4379) -> ()
                }
                frame 50 {
                  n3395 = local write "S 51"(w4380) -> ()
                }
                frame 51 {
                  n3396 = local write "S 52"(w4381) -> ()
                }
                frame 52 {
                  n3397 = local write "S 53"(w4382) -> ()
                }
                frame 53 {
                  n3398 = local write "S 54"(w4383) -> ()
                }
                frame 54 {
                  n3399 = local write "S 55"(w4384) -> ()
                }
                frame 55 {
                  n3400 = local write "S 56"(w4385) -> ()
                }
                frame 56 {
                  n3401 = local write "S 57"(w4386) -> ()
                }
                frame 57 {
                  n3402 = local write "S 58"(w4387) -> ()
                }
                frame 58 {
                  n3403 = local write "S 59"(w4388) -> ()
                }
                frame 59 {
                  n3404 = local write "S 60"(w4389) -> ()
                }
                frame 60 {
                  n3405 = local write "S 62"(w4390) -> ()
                }
                frame 61 {
                  n3406 = local write "S 63"(w4391) -> ()
                }
                frame 62 {
                  n3407 = local write "S 64"(w4392) -> ()
                }
                frame 63 {
                  n3408 = local write "S 65"(w4393) -> ()
                }
                frame 64 {
                  n3409 = local write "S 66"(w4394) -> ()
                }
                frame 65 {
                  n3410 = local write "S 67"(w4395) -> ()
                }
                frame 66 {
                  n3411 = local write "S 68"(w4396) -> ()
                }
                frame 67 {
                  n3412 = local write "S 69"(w4397) -> ()
                }
                frame 68 {
                  n3413 = local write "S 70"(w4398) -> ()
                }
                frame 69 {
                  n3414 = local write "S 71"(w4399) -> ()
                }
                frame 70 {
                  n3415 = local write "S 72"(w4400) -> ()
                }
                frame 71 {
                  n3416 = local write "S 73"(w4401) -> ()
                }
                frame 72 {
                  n3417 = local write "S 74"(w4402) -> ()
                }
                frame 73 {
                  n3418 = local write "S 75"(w4403) -> ()
                }
                frame 74 {
                  n3419 = local write "S 76"(w4404) -> ()
                }
                frame 75 {
                  n3420 = local write "S 77"(w4405) -> ()
                }
                frame 76 {
                  n3421 = local write "S 78"(w4406) -> ()
                }
                frame 77 {
                  n3422 = local write "S 79"(w4407) -> ()
                }
                frame 79 {
                  n3423 = property on="Sample Temperature ( °C )" class="XYGraph (strict)"("Y Scale.Name Label.Text"=w4408) -> ()  [unwired: 2 in, 2 out]
                }
                frame 80 {
                  n3424 = local write "S 81"(w4409) -> ()
                  n3425 = property on="Humidity ( %RH )" class="XYGraph (strict)"("Y Scale.Name Label.Text"=w4409) -> ()  [unwired: 2 in, 2 out]
                }
                frame 78 {
                  n3426 = property on="Air Temperature  ( °C )" class="XYGraph (strict)"("X Scale.Name Label.Text"=w4410) -> ()  [unwired: 2 in, 2 out]
                  n3427 = property on="Humidity ( %RH )" class="XYGraph (strict)"("X Scale.Name Label.Text"=w4410) -> ()  [unwired: 2 in, 2 out]
                  n3428 = property on="Sample Temperature ( °C )" class="XYGraph (strict)"("X Scale.Name Label.Text"=w4410) -> ()  [unwired: 2 in, 2 out]
                  n3429 = property on="Coefficient Of Friction" class="XYGraph (strict)"("X Scale.Name Label.Text"=w4410) -> ()  [unwired: 2 in, 2 out]
                }
                frame 81 {
                  n3430 = property on="Air Temperature  ( °C )" class="XYGraph (strict)"("Y Scale.Name Label.Text"=w4411) -> ()  [unwired: 2 in, 2 out]
                }
                frame 82 {
                  n3431 = local write "S 84"(w4412) -> ()
                }
                frame 83 {
                  n3432 = local write "S 85"(w4413) -> ()
                }
                frame 84 {
                  n3433 = local write "S 86"(w4414) -> ()
                }
                frame 85 {
                  n3434 = local write "S 87"(w4415) -> ()
                }
                frame 86 {
                  n3435 = local write "S 88"(w4416) -> ()
                }
                frame 87 {
                }
                frame 88 {
                  n3436 = local write "S 90"(w4418) -> ()
                }
                frame 89 {
                  n3437 = local write "S 91"(w4419) -> ()
                }
                frame 90 {
                  n3438 = local write "S 92"(w4420) -> ()
                }
                frame 91 {
                  n3439 = local write "S 93"(w4421) -> ()
                }
                frame 92 {
                  n3440 = local write "S 94"(w4422) -> ()
                }
                frame 93 {
                  n3441 = local write "S 95"(w4423) -> ()
                }
                frame 94 {
                  n3442 = local write "S 96"(w4424) -> ()
                }
                frame 95 {
                  n3443 = local write "S 97"(w4425) -> ()
                }
                frame 96 {
                  n3444 = local write "S 98"(w4426) -> ()
                }
                frame 97 {
                  n3445 = local write "S 99"(w4427) -> ()
                }
                frame 98 {
                  n3446 = local write "S 100"(w4428) -> ()
                }
                frame 99 {
                  n3447 = local write "S 101"(w4429) -> ()
                }
                frame 100 {
                  n3448 = local write "S 102"(w4430) -> ()
                }
                frame 101 {
                  n3449 = local write "S 103"(w4431) -> ()
                }
                frame 102 {
                  n3450 = local write "S 104"(w4432) -> ()
                }
                frame 103 {
                  n3451 = local write "S 105"(w4433) -> ()
                }
                frame 104 {
                  n3452 = local write "S 106"(w4434) -> ()
                }
                frame 105 {
                }
                frame 106 {
                  n3453 = property on="OK Button 17" class="Bool (strict)"("Boolean Text.Text"=w4435) -> ()  [unwired: 2 in, 2 out]
                }
                frame 107 {
                  n3454 = property on="OK Button 16" class="Bool (strict)"("Boolean Text.Text"=w4436) -> ()  [unwired: 2 in, 2 out]
                }
                frame 108 {
                  n3455 = property on="TITTLE" class="Str"("Caption.Text"=w4437) -> ()  [unwired: 2 in, 2 out]
                }
                frame 109 {
                  "String 30" <- w4438
                }
                frame 110 {
                  n3456 = property on="Test Date" class="Str"("Caption.Text"=w4439) -> ()  [unwired: 2 in, 2 out]
                  "String 31" <- w4439
                }
                frame 111 {
                  n3457 = property on="Sample ID" class="Str"("Caption.Text"=w4440) -> ()  [unwired: 2 in, 2 out]
                  "String 32" <- w4440
                }
                frame 112 {
                  n3458 = property on="Tested by" class="Str"("Caption.Text"=w4441) -> ()  [unwired: 2 in, 2 out]
                  "String 33" <- w4441
                }
                frame 113 {
                  n3459 = property on="System Configured Printers 2" class="Arr (strict)"("Caption.Text"=w4442) -> ()  [unwired: 2 in, 2 out]
                }
                frame 114 {
                  n3460 = property on="Selected Printer" class="Str"("Caption.Text"=w4443) -> ()  [unwired: 2 in, 2 out]
                }
                frame 115 {
                  n3461 = property on="Select Printer 3" class="DigNum (strict)"("Caption.Text"=w4444) -> ()  [unwired: 2 in, 2 out]
                }
                frame 116 {
                  n3462 = property on="Print" class="Bool (strict)"("Boolean Text.Text"=w4445) -> ()  [unwired: 2 in, 2 out]
                }
                frame 117 {
                  "String 41" <- w4446
                }
                frame 118 {
                  n3463 = property on="tested by" class="Str"("Caption.Text"=w4447) -> ()  [unwired: 2 in, 2 out]
                }
                frame 119 {
                }
                frame 120 {
                  n3464 = property on="Export" class="Bool (strict)"("Boolean Text.Text"=w4448) -> ()  [unwired: 2 in, 2 out]
                }
                frame 121 {
                  n3465 = property on="TEMP INTERCEPT:" class="DigNum (strict)"("Caption.Text"=w4449) -> ()  [unwired: 2 in, 2 out]
                }
                frame 122 {
                  n3466 = property on="AIR TEMP INTERCEPT:" class="DigNum (strict)"("Caption.Text"=w4450) -> ()  [unwired: 2 in, 2 out]
                }
                frame 123 {
                  n3467 = property on="Select File Type" class="Enum (strict)"("Caption.Text"=w4451) -> ()  [unwired: 2 in, 2 out]
                }
                frame 124 {
                  n3468 = property on="s.NO" class="Str"("Caption.Text"=w4452) -> ()  [unwired: 2 in, 2 out]
                  "String 45" <- w4452
                }
                frame 125 {
                  n3469 = property on="trip1 8" class="Bool (strict)"("Boolean Text.Text"=w4453) -> ()  [unwired: 2 in, 2 out]
                }
                frame 126, Default {
                }
              }
            }
          }
          frame #1 {
            w4461 = TRUE ("Visible")
            n3470 = local read "S 91"() -> (w4478:string)
            n3471 = local read "S 90"() -> (w4477:string)
            n3472 = local read "S 88"() -> (w4476:string)
            n3473 = property on="File Path" class="Path"("Caption.Text"=w4477) -> ()  [unwired: 2 in, 2 out]
            n3474 = property on="SrvM CP" class="Bool (strict)"("Boolean Text.Text"=w4476) -> ()  [unwired: 2 in, 2 out]
            n3475 = local read "S 71"() -> (w4471:string)
            n3476 = local read "S 86"() -> (w4473:string)
            n3477 = local read "S 85"() -> (w4474:string)
            n3478 = local read "S 87"() -> (w4472:string)
            n3479 = local read "S 84"() -> (w4475:string)
            n3480 = local read "S 103"() -> (w4460:string)
            n3481 = local read "S 104"() -> (w4459:string)
            n3482 = property on="ENTER THE NEW PASSWORD" class="Str"("Caption.Text"=w4472) -> ()  [unwired: 2 in, 2 out]
            n3483 = property on="Password" class="Str"("Caption.Text"=w4474) -> ()  [unwired: 2 in, 2 out]
            n3484 = property on="ENTER CURRENT PASSWORD" class="Str"("Caption.Text"=w4473) -> ()  [unwired: 2 in, 2 out]
            n3485 = property on="EDIT" class="Bool (strict)"("Boolean Text.Text"=w4471) -> ()  [unwired: 2 in, 2 out]
            n3486 = property on="SAVE" class="Bool (strict)"("Boolean Text.Text"=w4475) -> ()  [unwired: 2 in, 2 out]
            n3487 = Build Array(w4460, w4459) -> (w4458:string[])
            n3488 = property on="Heater Button" class="Bool (strict)"("Strings [4]"=w4458) -> ()  [unwired: 2 in, 2 out]
            n3489 = property on="CH-HUMIDITY WET" class="DigNum (strict)"("Caption.Size to Text?"=w4461) -> ()  [unwired: 2 in, 2 out]
            n3490 = property on="CH-HUMIDITY DRY" class="DigNum (strict)"("Caption.Size to Text?"=w4461) -> ()  [unwired: 2 in, 2 out]
            n3491 = property on="CH-POWER -" class="DigNum (strict)"("Caption.Size to Text?"=w4461) -> ()  [unwired: 2 in, 2 out]
            n3492 = property on="CH-HEATER" class="DigNum (strict)"("Caption.Size to Text?"=w4461) -> ()  [unwired: 2 in, 2 out]
            n3493 = property on="CH-POWER +" class="DigNum (strict)"("Caption.Size to Text?"=w4461) -> ()  [unwired: 2 in, 2 out]
            n3494 = local read "S 92"() -> (w4470:string)
            n3495 = local read "S 93"() -> (w4469:string)
            n3496 = local read "S 105"() -> (w4456:string)
            n3497 = local read "S 106"() -> (w4455:string)
            n3498 = Build Array(w4470, w4469) -> ()  [unwired: 1 out]
            n3499 = Build Array(w4456, w4455) -> (w4457:string[])
            n3500 = local read "S 95"() -> (w4467:string)
            n3501 = local read "S 94"() -> (w4468:string)
            n3502 = local read "bs"() -> (w4483:string)
            n3503 = local read "as"() -> (w4484:string)
            n3504 = property on="Humidity" class="Bool (strict)"("Strings [4]"=w4457) -> ()  [unwired: 2 in, 2 out]
            n3505 = Concatenate Strings(w4483, "\r", w4484) -> ()  [unwired: 1 out]
            n3506 = property on="STROKE GAIN :" class="DigNum (strict)"("Caption.Text"=w4467) -> ()  [unwired: 2 in, 2 out]
            n3507 = property on="DISPLACEMENT :" class="DigNum (strict)"("Caption.Text"=w4468) -> ()  [unwired: 2 in, 2 out]
            n3508 = property on="Rh After" class="DigNum (strict)"("Caption.Size to Text?"=TRUE ("Caption.Size to Text")) -> ()  [unwired: 2 in, 2 out]
            n3509 = local read "S 48"() -> (w4507:string)
            n3510 = local read "S 50"() -> (w4505:string)
            n3511 = local read "S 51"() -> (w4504:string)
